vi "LUnit Init.vi"(8 "error in (no error)":errorcluster, 11 "Coverage Report In":refnum<class "Coverage Report.lvclass">) -> (0 "error out":errorcluster, 3 "Coverage Report Out":refnum<class "Coverage Report.lvclass">)   [LabVIEW 2020, in "Coverage Report.lvclass"]
uses:
  Coverage Report.lvclass
  Coverage Report.lvclass/Coverage Report.ctl
  <vilib>/Astemes/LUnit/Framework/LUnit Configuration Manager.lvclass
  <vilib>/Astemes/LUnit/Framework/LUnit Paths.lvlib
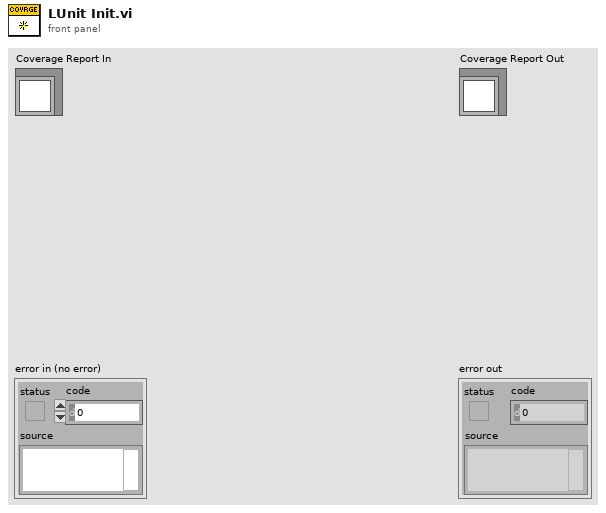
[diagram p1: front panel]
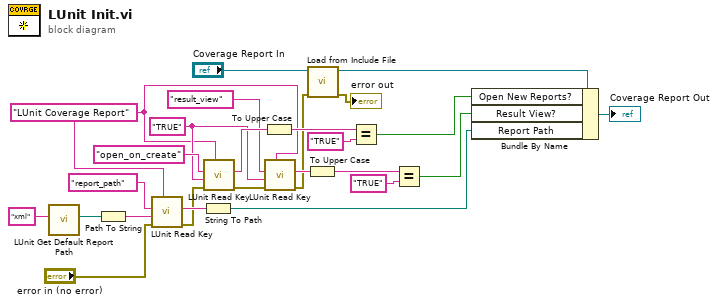
[diagram p0: block diagram]
diagram:
  w9 = "TRUE" ("y")
  w8 = "LUnit Coverage Report"
  n1 = call <vilib>:"LUnit Get Default Report Path.vi"("File Extension"="xml") -> ("Default Report Directory"=w14:path)  [unwired: 9 in, 1 out]
  n2 = Path To String(path=w14) -> (string=w21:string)
  n3 = call <vilib>:"LUnit Read Key.vi"("section"=w8, "error in (no error)"="error in (no error)", "default value"=w21, "key"="report_path" ("Name")) -> ("error out"=w19:errorcluster, "value"=w20:string)  [unwired: 6 in]
  n4 = String To Path(string=w20) -> (path=w13:path)
  n5 = call <vilib>:"LUnit Read Key.vi"("section"=w8, "error in (no error)"=w19, "default value"=w9, "key"="open_on_create" ("Name")) -> ("error out"=w2:errorcluster, "value"=w16:string)  [unwired: 6 in]
  n6 = To Upper Case(1:w16) -> (0:w26:string)
  n7 = call <vilib>:"LUnit Read Key.vi"("section"=w8, "error in (no error)"=w2, "default value"=w9, "key"="result_view") -> ("error out"=w1:errorcluster, "value"=w4:string)  [unwired: 6 in]
  n8 = To Upper Case(1:w4) -> (0:w5:string)
  n9 = call "Load from Include File.vi"("error in (no error)"=w1, "Coverage Report in"="Coverage Report In") -> ("error out"=→"error out":errorcluster, "Coverage Report out"=w11:refnum<class "Coverage Report.lvclass">)  [unwired: 8 in]
  n10 = Equal?(x=w26, y="TRUE") -> (x = y?=w24:bool)
  n11 = Equal?(x=w5, y="TRUE") -> (x = y?=w3:bool)
  n12 = Bundle By Name(cluster=w11, "Open New Reports?"=w24, "Result View?"=w3, "Report Path"=w13) -> (→"Coverage Report Out":refnum<class "Coverage Report.lvclass">)
